vi "varXNode_Mutate_8_1_0_0.vi"(8 "error in (no error)":errorcluster, 9 "Replies in":string[](array[string]), 10 "Version":T1, 11 "Old State":variant) -> (0 "error out":errorcluster, 1 "Replies out":string[](array[string]), 2 "Version Out":T1, 3 "New State":variant)   [LabVIEW 2017, in "varXNode.xnode"]
uses:
  <vilib>/variable/varXNode.llb/varXNode.xnode
  <vilib>/XNodeSupport/XNodeVersion.ctl
  <vilib>/XNodeSupport/XNodeUShort.ctl
  <vilib>/variable/varXNode.llb/varXNode_old_1_0_0_6.ctl
  <vilib>/variable/Type Descriptor.ctl
  <vilib>/variable/varXNode.llb/varXNode_old_8_1_0_0.ctl
  <vilib>/XNodeSupport/NI_XNodeSupport.lvlib
  <vilib>/variable/NI_Variable.lvlib
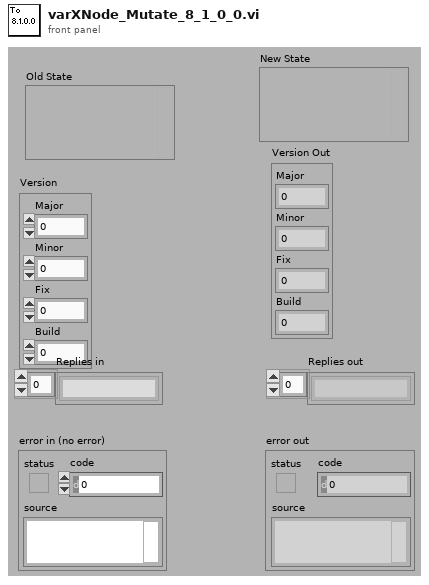
[diagram p1: front panel]
types:
  T1 = typedef "NI_XNodeSupport.lvlib/XNodeVersion.ctl" = cluster{"Major":T2, "Minor":T2, "Fix":T2, "Build":T2}
  T2 = typedef "NI_XNodeSupport.lvlib/XNodeUShort.ctl" = u16
  T3 = typedef "varXNode.xnode/varXNode_old_8_1_0_0.ctl" = cluster{"Write":bool, "ShowTimestamp":bool, "CachedName":string, "CachedTypeDesc":T4, "CachedFeaturePacks":string[], "Custom Rule":string, "ProjectPath":string, "Bad Code":bool, "ContextName":string, "Allow Timestamp":bool}
  T4 = typedef "NI_Variable.lvlib/Type Descriptor.ctl" = cluster{"Variant":variant}
  T5 = typedef "varXNode.xnode/varXNode_old_1_0_0_6.ctl" = cluster{"Write":bool, "ShowTimestamp":bool, "CachedName":string, "CachedTypeDesc":T4, "CachedFeaturePacks":string[], "Custom Rule":string, "ProjectPath":string, "Bad Code":bool, "ContextName":string}
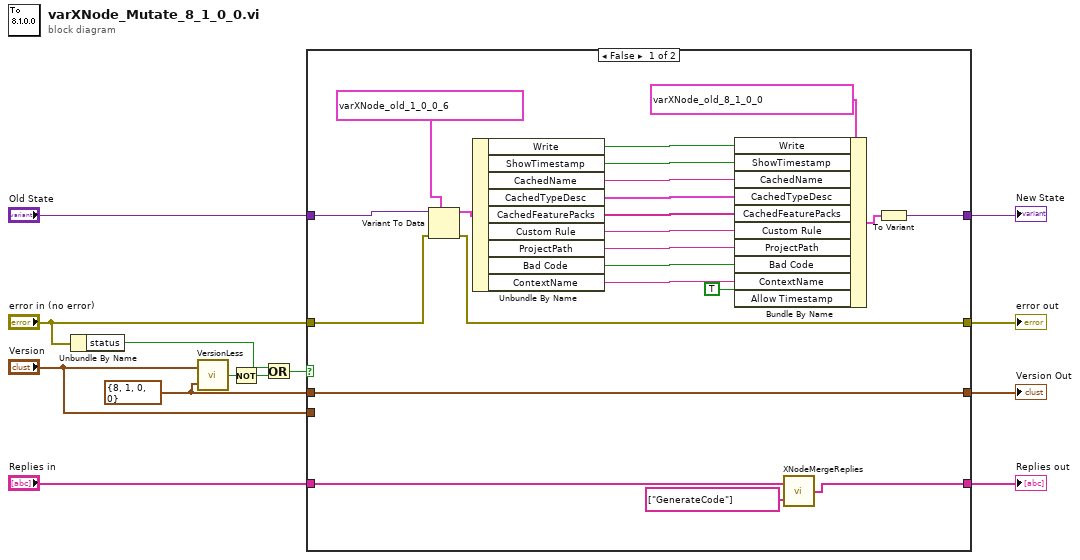
[diagram p0: block diagram]
diagram:
  w12 = T1 {"Major"=8, "Minor"=1, "Fix"=0, "Build"=0} ("y")
  n1 = Unbundle By Name("error in (no error)") -> ("status"=w4:bool)
  n2 = call <vilib>:"VersionLess.vi"("y"=w12, "x"="Version") -> ("x < y?"=w13:bool)
  n3 = Not(x=w13) -> (.not. x?=w3:bool)
  n4 = Or(x=w4, y=w3) -> (x .or. y?=w6:bool)
  n5 = case shown="False" w6 {
    tunnel: w12 -> [w35 _]
    tunnel: [w32 w39] -> w11
    tunnel: "Old State" -> [w34 w39]
    tunnel: [w35 w38] -> w9
    tunnel: "Version" -> [_ w38]
    tunnel: [w17 w37] -> w7
    tunnel: "error in (no error)" -> [w18 w37]
    tunnel: [w14 w36] -> w2
    tunnel: "Replies in" -> [w15 w36]
    frame False {
      n6 = Variant To Data(error in=w18, type=T5 {"Write"=FALSE, "ShowTimestamp"=FALSE, "CachedName"="", "CachedTypeDesc"={"Variant"=variant}, "CachedFeaturePacks"=[], "Custom Rule"="", "ProjectPath"="", "Bad Code"=FALSE, "ContextName"=""} ("State"), Variant=w34) -> (data=w33:T5, error out=w17:errorcluster)
      n7 = Unbundle By Name(w33) -> ("Write"=w28:bool, "ShowTimestamp"=w27:bool, "CachedName"=w26:string, "CachedTypeDesc"=w25:T4, "CachedFeaturePacks"=w24:string[], "Custom Rule"=w23:string, "ProjectPath"=w22:string, "Bad Code"=w21:bool, "ContextName"=w20:string)
      n8 = Bundle By Name(cluster=T3 {"Write"=FALSE, "ShowTimestamp"=FALSE, "CachedName"="", "CachedTypeDesc"={"Variant"=variant}, "CachedFeaturePacks"=[], "Custom Rule"="", "ProjectPath"="", "Bad Code"=FALSE, "ContextName"="", "Allow Timestamp"=FALSE} ("State"), "Write"=w28, "ShowTimestamp"=w27, "CachedName"=w26, "CachedTypeDesc"=w25, "CachedFeaturePacks"=w24, "Custom Rule"=w23, "ProjectPath"=w22, "Bad Code"=w21, "ContextName"=w20, "Allow Timestamp"=TRUE) -> (w29:T3)
      n9 = call <vilib>:"XNodeMergeReplies.vi"("New Replies"=string[] ["GenerateCode"] ("Replies out"), "Old Replies"=w15) -> ("Merged Replies"=w14:string[])
      n10 = To Variant(anything=w29) -> (Variant=w32:variant)
    }
    frame True {
      # "Either there was an error in,\nor the version is not less than 1.0.0.6.\nPass input values out."
    }
  }
  "New State" <- w11
  "Version Out" <- w9
  "error out" <- w7
  "Replies out" <- w2
